vi "Home Call Cylender.vi"(9 "Enum":T1(ring)) -> ()   [LabVIEW 2020]
uses:
  Galobal variable_TI.vi
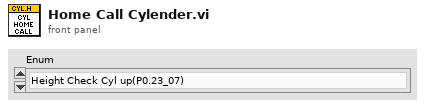
[diagram p1: front panel]
types:
  T1 = enum16{"Height Check Cyl up(P0.23_07)", "Height Check Cyl  Up RS_(AI12_26)", "Height Check Cyl  Dn RS_(AI13_27)", "Height Check Cyl dn(P0.24_08)", "Camera Cyl Rev(P0.26_10)", "Camera Cyl fwd(P0.25_09)", "Height Check Cyl off", "Camera Cyl Rev_RS(AI15_29)", "Camera Cyl off", "Camera Cyl FWD_RS(AI14_28)", "LCD Rotation Dn(P0.28_12)", "LCD Rotation dn proxi(AI17_31)", "LCD Rotation Up(P0.27_11)", "LCD Rotation dn proxi(AI16_30)"}
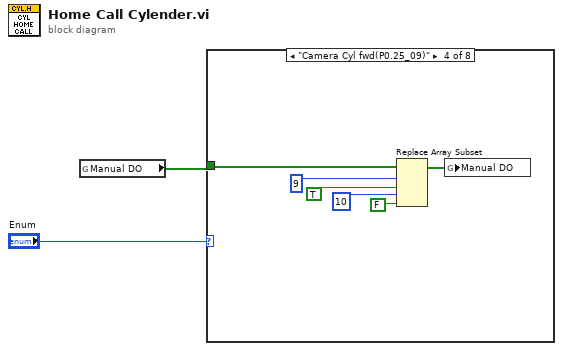
[diagram p0: block diagram]
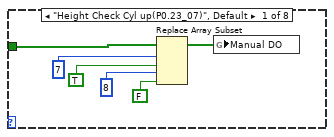
[diagram p2: hidden frame]
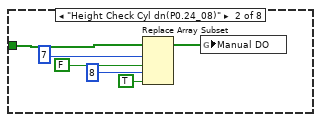
[diagram p3: hidden frame]
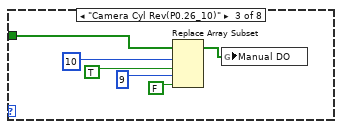
[diagram p4: hidden frame]
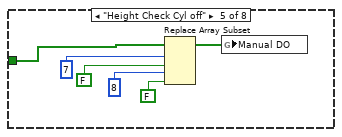
[diagram p5: hidden frame]
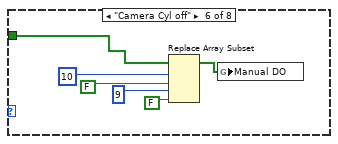
[diagram p6: hidden frame]
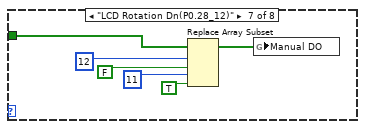
[diagram p7: hidden frame]
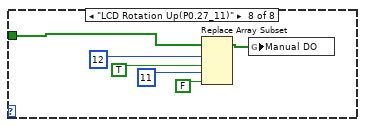
[diagram p8: hidden frame]
diagram:
  n1 = global read "Galobal variable_TI.vi" "Manual DO"() -> (w2:bool[])
  n2 = case shown="\"Camera Cyl fwd(P0.25_09)\"" "Enum" {
    tunnel: w2 -> [w7 w10 w16 w22 w27 w33 w40 w46]
    frame "Height Check Cyl up(P0.23_07)", Default {
      n3 = Replace Array Subset(array=w7, new element #1=TRUE ("new element/subarray"), index #1=7 ("index"), new element #2=FALSE ("new element/subarray"), index #2=8 ("index")) -> (w3:bool[])
      n4 = global write "Galobal variable_TI.vi" "Manual DO"(w3) -> ()
    }
    frame "Height Check Cyl dn(P0.24_08)" {
      n5 = Replace Array Subset(array=w10, new element #1=FALSE ("new element/subarray"), index #1=7 ("index"), new element #2=TRUE ("new element/subarray"), index #2=8 ("index")) -> (w9:bool[])
      n6 = global write "Galobal variable_TI.vi" "Manual DO"(w9) -> ()
    }
    frame "Camera Cyl Rev(P0.26_10)" {
      n7 = Replace Array Subset(array=w16, new element #1=TRUE ("new element/subarray"), index #1=10 ("index"), new element #2=FALSE ("new element/subarray"), index #2=9 ("index")) -> (w15:bool[])
      n8 = global write "Galobal variable_TI.vi" "Manual DO"(w15) -> ()
    }
    frame "Camera Cyl fwd(P0.25_09)" {
      n9 = Replace Array Subset(array=w22, new element #1=TRUE ("new element/subarray"), index #1=9 ("index"), new element #2=FALSE ("new element/subarray"), index #2=10 ("index")) -> (w21:bool[])
      n10 = global write "Galobal variable_TI.vi" "Manual DO"(w21) -> ()
    }
    frame "Height Check Cyl off" {
      n11 = Replace Array Subset(array=w27, new element #1=FALSE ("new element/subarray"), index #1=7 ("index"), new element #2=FALSE ("new element/subarray"), index #2=8 ("index")) -> (w28:bool[])
      n12 = global write "Galobal variable_TI.vi" "Manual DO"(w28) -> ()
    }
    frame "Camera Cyl off" {
      n13 = Replace Array Subset(array=w33, new element #1=FALSE ("new element/subarray"), index #1=10 ("index"), new element #2=FALSE ("new element/subarray"), index #2=9 ("index")) -> (w34:bool[])
      n14 = global write "Galobal variable_TI.vi" "Manual DO"(w34) -> ()
    }
    frame "LCD Rotation Dn(P0.28_12)" {
      n15 = Replace Array Subset(array=w40, new element #1=FALSE ("new element/subarray"), index #1=12 ("index"), new element #2=TRUE ("new element/subarray"), index #2=11 ("index")) -> (w39:bool[])
      n16 = global write "Galobal variable_TI.vi" "Manual DO"(w39) -> ()
    }
    frame "LCD Rotation Up(P0.27_11)" {
      n17 = Replace Array Subset(array=w46, new element #1=TRUE ("new element/subarray"), index #1=12 ("index"), new element #2=FALSE ("new element/subarray"), index #2=11 ("index")) -> (w45:bool[])
      n18 = global write "Galobal variable_TI.vi" "Manual DO"(w45) -> ()
    }
  }
